vi "Array of VData to VCluster.vi"(8 "error in (no error)":errorcluster, 9 "Cluster Name":string, 10 "Array":refnum<class "variant.lvclass">[](array[class])) -> (0 "error out":errorcluster, 2 "VCluster":refnum<class "variant.lvclass">)   [LabVIEW 2020, in "variant.lvlib" / "variant.lvclass"]
doc: "Returns the elements of an array as elements of a variant cluster."
uses:
  Type Descriptor Enumeration.ctl
  variant.lvclass
  variant.lvclass/variant.ctl
  openg_variant.lvlib
  Type Descriptor/TD.lvclass
  Bytes/Bytes.lvclass
  DataString/DataString.lvclass
  C:/projects/OpenG-Variant-Data-Library/source/library/Bytes/Bytes.lvclass
  C:/projects/OpenG-Variant-Data-Library/source/library/LVData/DataString/DataString.lvclass
panel:
  # "[OpenG VI Tags] ***Do Not Remove***"
  # "Array of VData to VCluster.vi\n\nReturns the elements of an array as elements of a variant cluster.\n\nPlease visit http://www.OpenG.org to learn about the\nOpen Source LabVIEW software movement.\n\nNOTICE -- YOU MUST LEAVE THIS NOTICE IN PLACE.  PER THE TERMS OF THE LICENSE BELOW, YOU MAY SUBLICENSE THIS SOFTWARE \nIN ANY WAY THAT DOES NOT CONFLICT WITH THIS LICENSE.\n\n### BSD License (http://www.opensource.org/licenses/bsd-license.php) Begin ###\n \nCopyright (c) 2002, Jean-Pierre Drolet <drolet_jp@hotmail.com>\nCopyright (c) 2002-2006, Jim Kring <jim@jimkring.com>\n\nAll rights reserved.\n\nRedistribution and use in source and binary forms, with or without modification, are permitted provided that the following conditions are met:\n\n    * Redistributions of source code must retain the above copyright notice, this list of conditions and the following disclaimer.\n    * Redistributions in binary form must reproduce the above copyright notice, this list of conditions and the following disclaimer in the \n       documentation and/or other materials provided with the distribution.\n    * Neither the name of SciWare, James Kring, Inc., nor the names of its contributors may be used to endorse or promote products derived \n       from this software without specific prior written permission.\n\nTHIS SOFTWARE IS PROVIDED BY THE COPYRIGHT HOLDERS AND CONTRIBUTORS \"AS IS\" AND ANY EXPRESS OR IMPLIED WARRANTIES, \nINCLUDING, BUT NOT LIMITED TO, THE IMPLIED WARRANTIES OF MERCHANTABILITY AND FITNESS FOR A PARTICULAR PURPOSE ARE \nDISCLAIMED. IN NO EVENT SHALL THE COPYRIGHT OWNER OR CONTRIBUTORS BE LIABLE FOR ANY DIRECT, INDIRECT, INCIDENTAL,\n SPECIAL, EXEMPLARY, OR CONSEQUENTIAL DAMAGES (INCLUDING, BUT NOT LIMITED TO, PROCUREMENT OF SUBSTITUTE GOODS OR \nSERVICES; LOSS OF USE, DATA, OR PROFITS; OR BUSINESS INTERRUPTION) HOWEVER CAUSED AND ON ANY THEORY OF LIABILITY, \nWHETHER IN CONTRACT, STRICT LIABILITY, OR TORT (INCLUDING NEGLIGENCE OR OTHERWISE) ARISING IN ANY WAY OUT OF THE USE \nOF THIS SOFTWARE, EVEN IF ADVISED OF THE POSSIBILITY OF SUCH DAMAGE.\n\n### BSD License End ###"
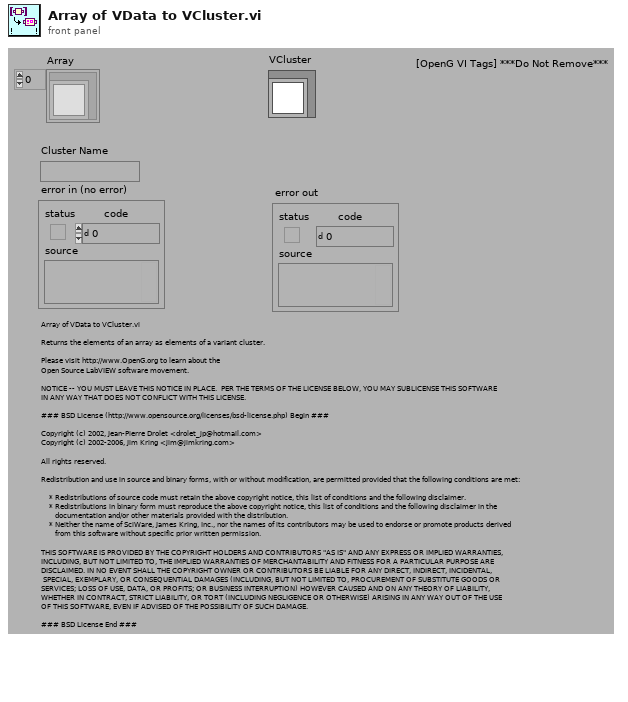
[diagram p1: front panel]
types:
  T1 = typedef "openg_variant.lvlib/Type Descriptor Enumeration.ctl" = enum8{"<Null>", "I8", "I16", "I32", "I64", "U8", "U16", "U32", "U64", "SGL", "DBL", "EXT", "CSG", "CDB", "CXT", "0x0F", "0x10", "0x11", "0x12", "0x13", "0x14", "Enum U8", "Enum U16", "Enum U32", "Enum U64", "SGL PQ", "DBL PQ", "EXT PQ", "CSG PQ", "CDB PQ", "CXT PQ", "0x1F", "0x20", "Boolean", "0x22", "0x23", "0x24", "0x25", "0x26", "0x27", "0x28", "0x29", "0x2A", "0x2B", "0x2C", "0x2D", "0x2E", "0x2F", "String", "0x31", "Path", "Pict", "0x34", "0x35", "0x36", "DAQ", "0x38", "0x39", "0x3A", "0x3B", "0x3C", "0x3D", "0x3E", "0x3F", "Array", "0x41", "0x42", "0x43", "0x44", "0x45", "0x46", "0x47", "0x48", "0x49", "0x4A", "0x4B", "0x4C", "0x4D", "0x4E", "0x4F", "Cluster", "0x51", "0x52", "Variant", "Waveform", "0x55", "0x56", "0x57", "0x58", "0x59", "0x5A", "0x5B", "0x5C", "0x5D", "0x5E", "Fixed Point", "0x60", "0x61", "0x62", "0x63", "0x64", "0x65", "0x66", "0x67", "0x68", "0x69", "0x6A", "0x6B", "0x6C", "0x6D", "0x6E", "0x6F", "Refnum", "0x71", "0x72", "Set Collection", "Map Collection"}
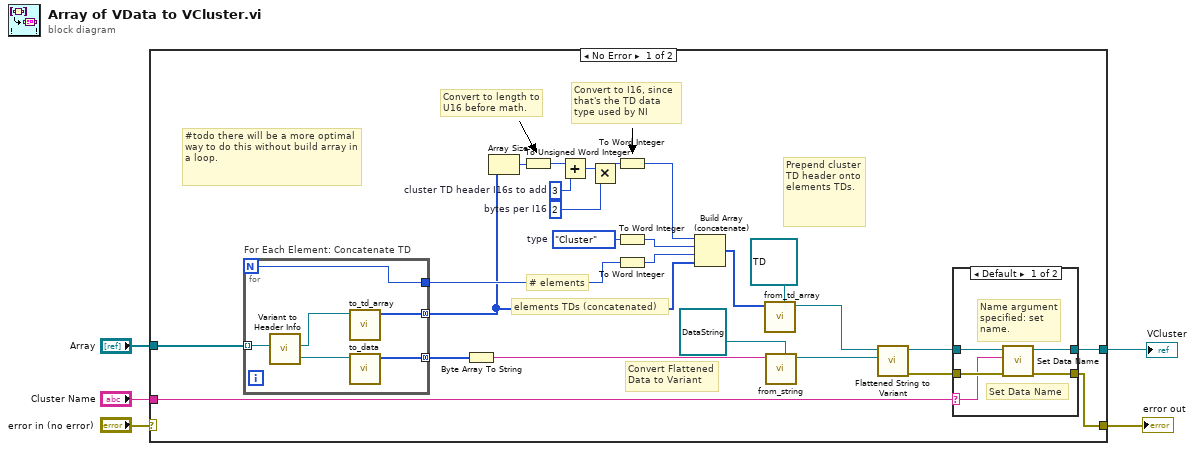
[diagram p0: block diagram]
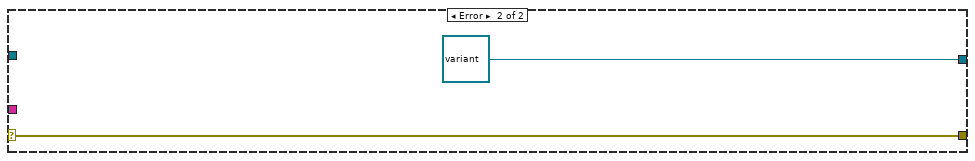
[diagram p3: hidden frame]
diagram:
  n1 = case shown="No Error" "error in (no error)" {
    selector: "error in (no error)" -> [_ w45]
    tunnel: [w23 w45] -> w5
    tunnel: [w24 refnum<class "variant.lvclass"> refnum ("variant out")] -> w1
    tunnel: "Array" -> [w26 _]
    tunnel: "Cluster Name" -> [w25 _]
    frame No Error {
      w18 = u16 2  # bytes per I16
      w20 = u16 3  # cluster TD header I16s to add
      w28 = Type_Descriptor_Enumeration."Cluster"  # type
      # "#todo there will be a more optimal way to do this without build array in a loop."
      # "Convert Flattened Data to Variant"
      # "elements TDs (concatenated)"
      # "Convert to length to U16 before math."
      # "Convert to I16, since that's the TD data type used by NI"
      # "Prepend cluster TD header onto elements TDs."
      # "# elements"
      n2 = for "For Each Element: Concatenate TD" {
        N -> [w42]
        tunnel: w26 -> [w43] mode=indexing
        tunnel: [w38] -> w14 mode=concatenating
        tunnel: [w42] -> w21
        tunnel: [w40] -> w15 mode=concatenating
        n3 = call "Variant to Header Info.vi"("Variant"=w43) -> ("TypeDescriptor"=w41:refnum<class "TD.lvclass">, "DataString"=w39:refnum<class "DataString.lvclass">)  [unwired: 3 in, 1 out]
        n4 = call "to_td_array.vi"("TypeDescriptor in"=w41) -> ("type string"=w40:i16[])  [unwired: 10 in]
        n5 = call "to_data.vi"("Bytes in"=w39) -> ("byte array"=w38:u8[])  [unwired: 10 in]
      }
      n6 = Byte Array To String(unsigned byte array=w14) -> (string=w12:string)
      n7 = Array Size(array=w15) -> (size(s)=w30:i32)
      n8 = To Unsigned Word Integer(number=w30) -> (unsigned 16bit integer=w17:u16)
      n9 = Add(x=w17, y=w20) -> (x+y=w19:u16)
      n10 = Multiply(x=w19, y=w18) -> (x*y=w16:u16)
      n11 = To Word Integer(number=w16) -> (16bit integer=w29:i16)
      n12 = To Word Integer(number=w28) -> (16bit integer=w22:i16)
      n13 = To Word Integer(number=w21) -> (16bit integer=w27:i16)
      n14 = Build Array (concatenate)(w29, w22, w27, w15) -> (w13:i16[])
      n15 = call "from_td_array.vi"("type"=refnum<class "TD.lvclass"> refnum, "type descriptor array"=w13) -> ("TypeDescriptor out"=w9:refnum<class "TD.lvclass">)  [unwired: 8 in, 1 out]
      n16 = call "from_string.vi"("type"=refnum<class "DataString.lvclass"> refnum ("DataString"), "string_data"=w12) -> ("Bytes out"=w8:refnum<class "DataString.lvclass">)  [unwired: 9 in]
      n17 = call "Flattened String to Variant.vi"("data"=w8, "type"=w9) -> ("error out"=w6:errorcluster, "variant out"=w7:refnum<class "variant.lvclass">)  [unwired: 8 in]
      n18 = case shown="Default" w25 {
        selector: w25 -> [w33 _]
        tunnel: [w31 w37] -> w24
        tunnel: w7 -> [w32 w37]
        tunnel: [w34 w36] -> w23
        tunnel: w6 -> [w35 w36]
        frame Default {
          # "Set Data Name"
          # "Name argument specified: set name."
          n19 = call "Set Data Name.vi"("error in (no error)"=w35, "Data Name"=w33, "LVData in"=w32) -> ("error out"=w34:errorcluster, "LVData out"=w31:refnum<class "variant.lvclass">)  [unwired: 7 in]
        }
        frame "" {
          # "Name argument is empty: don't set name."
        }
      }
    }
    frame Error {
    }
  }
  "error out" <- w5
  "VCluster" <- w1
